vi "Core Pre Launch Init.vi"(8 "error in (no error)":errorcluster, 11 "Sequencer Core in":refnum<class "Sequencer Core.lvclass">) -> (0 "error out":errorcluster, 3 "Sequencer Core out":refnum<class "Sequencer Core.lvclass">)   [LabVIEW 2020, in "Sequencer.lvlib" / "Sequencer Core.lvclass"]
doc: "This VI is executed during the Launch of the Sequencer Core. This will be executed during the Pre launch init phase of the Sequencer Actor.\n\nBy default this VI does nothing."
uses:
  Sequencer Core.lvclass
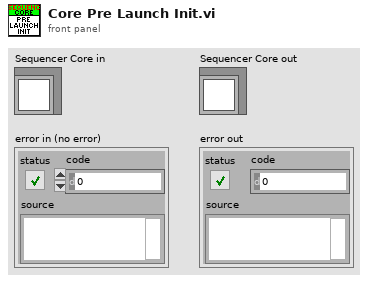
[diagram p1: front panel]
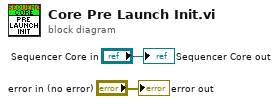
[diagram p0: block diagram]
diagram:
  "error out" <- "error in (no error)"
  "Sequencer Core out" <- "Sequencer Core in"
